vi "Time 4-2.vi"() -> ()   [LabVIEW 2022 SP3]
panel:
  out "x-y":dbl
  out "sum":i32
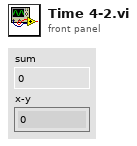
[diagram p1: front panel]
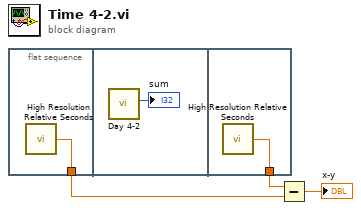
[diagram p0: block diagram]
diagram:
  n1 = flat-sequence {
    tunnel: [w4] -> w2
    tunnel: [w6] -> w3
    frame #0 {
      n2 = call <vilib>:"High Resolution Relative Seconds.vi"() -> ("relative seconds"=w4:dbl)
    }
    frame #1 {
      n3 = call "Day 4-2.vi"() -> ("sum"=→"sum":i32)  [unwired: 11 in]
    }
    frame #2 {
      n4 = call <vilib>:"High Resolution Relative Seconds.vi"() -> ("relative seconds"=w6:dbl)
    }
  }
  n5 = Subtract(x=w3, y=w2) -> (x-y=→"x-y":dbl)
